vi "Relays_FGV.vi"(5 "Akcija":T1, 6 "error in (no error)":errorcluster, 7 "ON/OFF":bool, 8 "Relay Number":u8, 9 "Input":u8[](array[numeric])) -> (0 "error out":errorcluster, 3 "Output":u8[](array[numeric]))   [LabVIEW 2020]
uses:
  Custom Ctls/Akcija.ctl
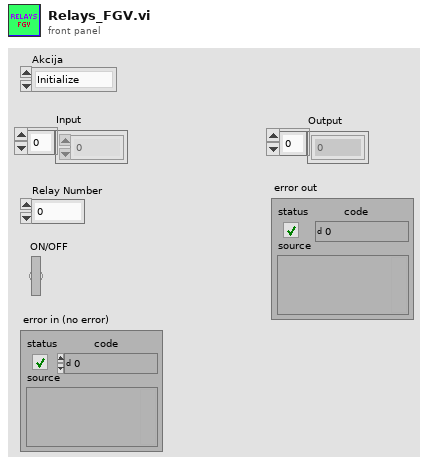
[diagram p1: front panel]
types:
  T1 = typedef "Akcija.ctl" = enum16{"Initialize", "Write", "Read", "Update"}
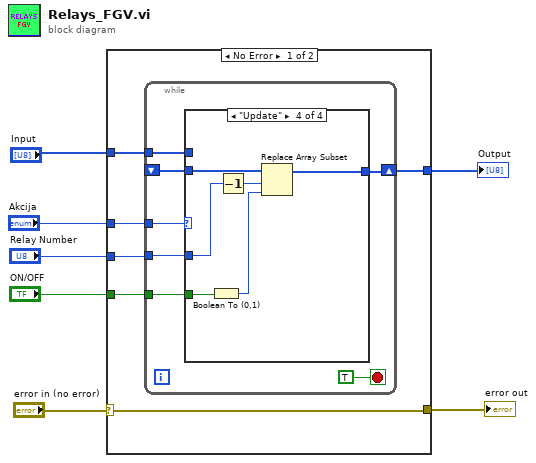
[diagram p0: block diagram]
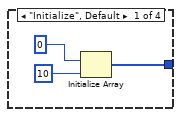
[diagram p2: hidden frame]
diagram:
  n1 = case shown="No Error" "error in (no error)" {
    selector: "error in (no error)" -> [w8 w33]
    tunnel: "Akcija" -> [w13 _]
    tunnel: [w8 w33] -> w5
    tunnel: "Input" -> [w11 w32]
    tunnel: [w12 w32] -> w3
    tunnel: "Relay Number" -> [w10 _]
    tunnel: "ON/OFF" -> [w9 _]
    frame No Error {
      n2 = while {
        tunnel: w13 -> [w19]
        shift-right: [w18] -> w12
        shift-left: _ -> [w16]
        tunnel: w11 -> [w17]
        tunnel: w10 -> [w15]
        tunnel: w9 -> [w14]
        stop <- TRUE stop-if-true
        n3 = case shown="\"Update\"" w19 {
          tunnel: [w23 w24 w25 w30] -> w18
          tunnel: w17 -> [_ w24 _ _]
          tunnel: w16 -> [_ _ w25 w26]
          tunnel: w15 -> [_ _ _ w31]
          tunnel: w14 -> [_ _ _ w27]
          frame "Initialize", Default {
            n4 = Initialize Array(u8 0, 10 ("dimension size")) -> (w23:u8[])
          }
          frame "Write" {
          }
          frame "Read" {
          }
          frame "Update" {
            n5 = Boolean To (0,1)(Boolean=w27) -> (0, 1=w28:i16)
            n6 = Decrement(x=w31) -> (x-1=w29:u8)
            n7 = Replace Array Subset(array=w26, new element=w28, index=w29) -> (w30:u8[])
          }
        }
      }
    }
    frame Error {
    }
  }
  "error out" <- w5
  "Output" <- w3
